vi "TM process commands.vi"(7 "Array in":T1[](array[typedef]) {"Time stamp" format="%<%H:%M:%S\n%Y/%m/%d>T"}, 8 "error in (no error)":errorcluster, 9 "Data":variant, 10 "Command":T2, 11 "Temperature monitor status in":T3 {"Last update" format="%<%H:%M:%S\n%y/%m/%d>T"}) -> (0 "error out":errorcluster, 1 "End?":bool, 2 "Array out":T1[](array[typedef]) {"Time stamp" format="%<%H:%M:%S\n%Y/%m/%d>T"}, 3 "Temperature monitor status out":T3 {"Last update" format="%<%H:%M:%S\n%y/%m/%d>T"})   [LabVIEW 2021, in "Temperature monitor.lvlib"]
uses:
  Temperature monitor.lvlib
  Typedefs/TM_status.ctl
  <userlib>/MatS Libs/MatS Mailman/TypeDefs/Mailbox ref.ctl
  Typedefs/TM_commands.ctl
  Typedefs/TM_sensors.ctl
  <userlib>/MatS Libs/MatS Libs.lvlib
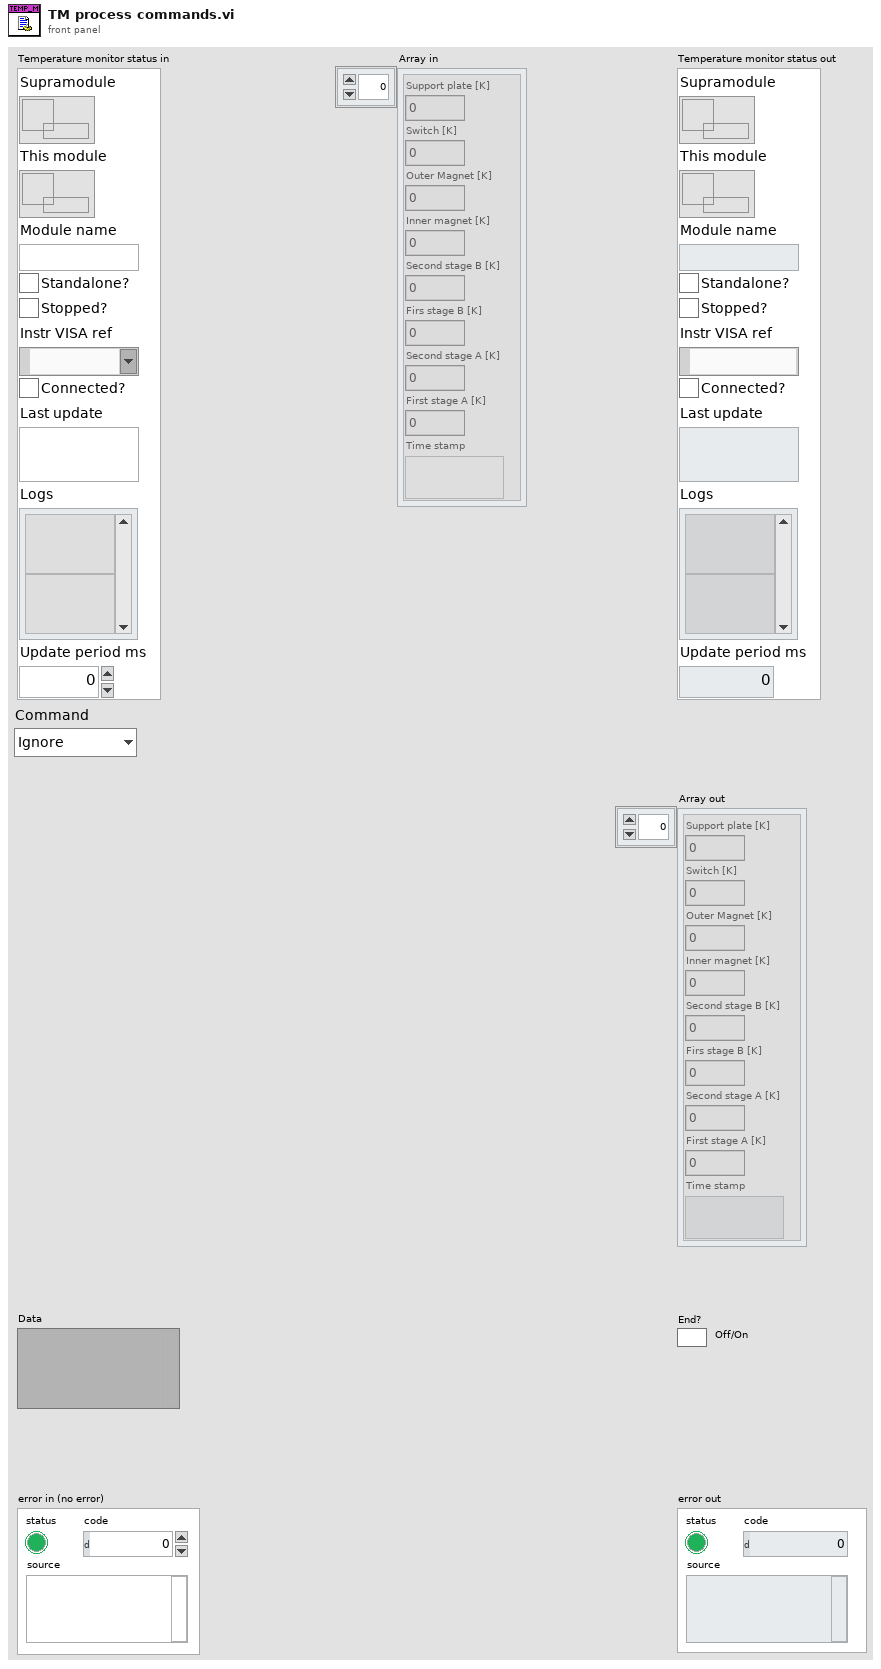
[diagram p1: front panel]
types:
  T1 = typedef "Temperature monitor.lvlib/TM_sensors.ctl" = cluster{"Support plate [K]":dbl, "Switch [K]":dbl, "Outer Magnet [K]":dbl, "Inner magnet [K]":dbl, "Second stage B [K]":dbl, "Firs stage B [K]":dbl, "Second stage A [K]":dbl, "First stage A [K]":dbl, "Time stamp":timestamp}
  T2 = typedef "Temperature monitor.lvlib/TM_commands.ctl" = enum16{"Ignore", "Log", "Connect", "Set timeout", "Update", "Disconnect", "End"}
  T3 = typedef "Temperature monitor.lvlib/TM_status.ctl" = cluster{"Supramodule":T4, "This module":T4, "Module name":string, "Standalone?":bool, "Stopped?":bool, "Instr VISA ref":refnum<visa-resource-name>, "Connected?":bool, "Last update":timestamp, "Logs":string[], "Update period ms":u32}
  T4 = typedef "MatS Libs.lvlib/Mailbox ref.ctl" = refnum<queue>
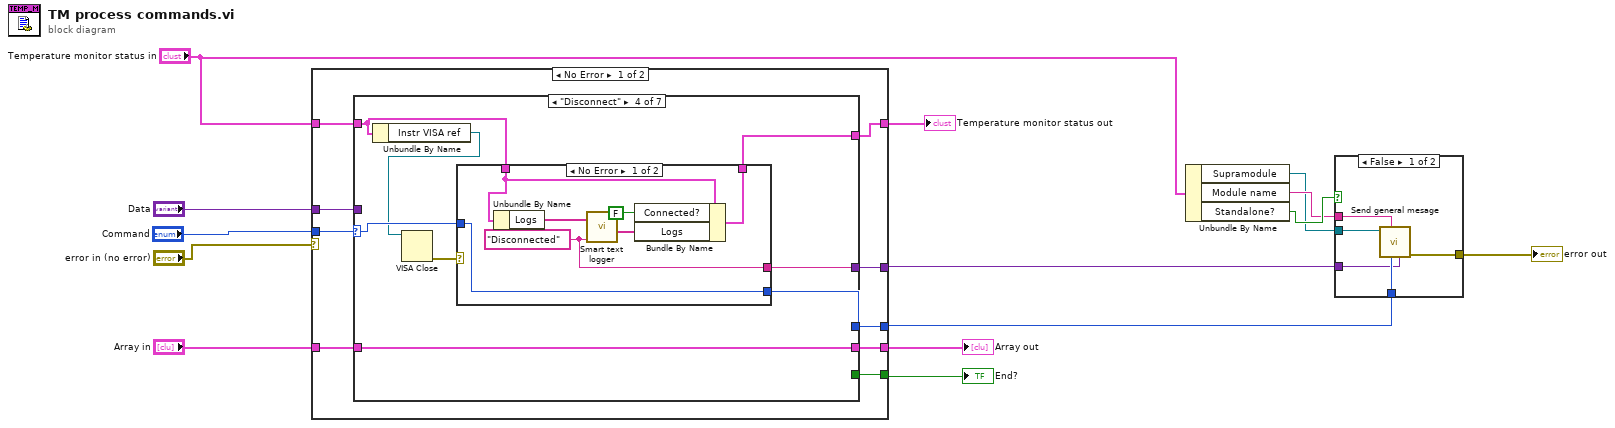
[diagram p0: block diagram]
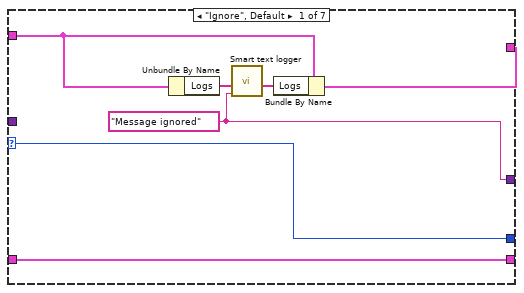
[diagram p2: hidden frame]
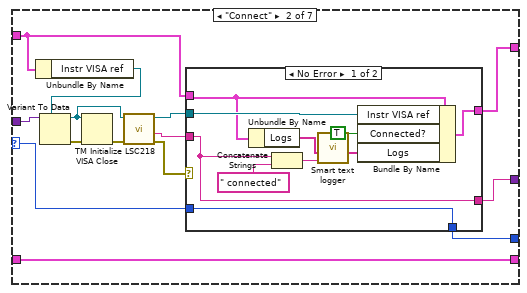
[diagram p3: hidden frame]
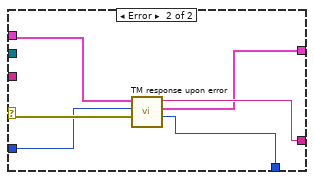
[diagram p4: hidden frame]
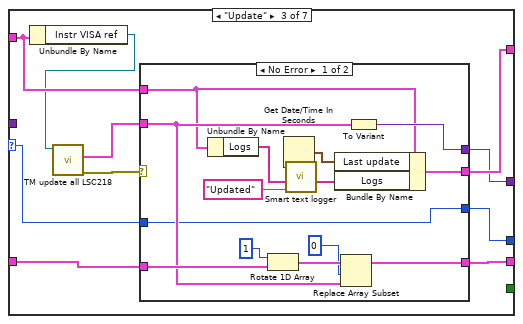
[diagram p5: hidden frame]
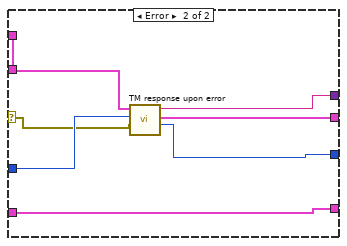
[diagram p6: hidden frame]
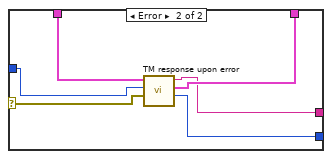
[diagram p7: hidden frame]
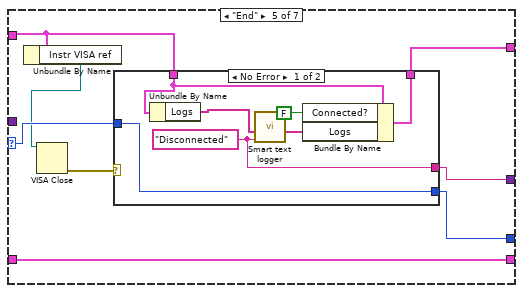
[diagram p8: hidden frame]
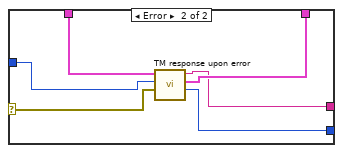
[diagram p9: hidden frame]
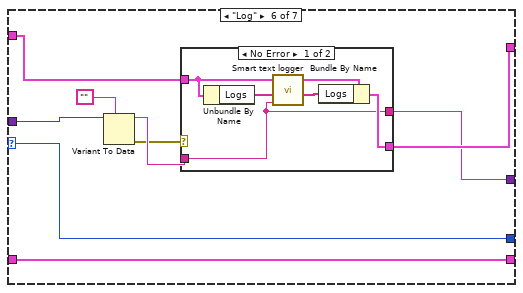
[diagram p10: hidden frame]
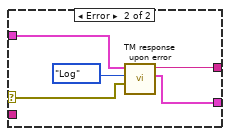
[diagram p11: hidden frame]
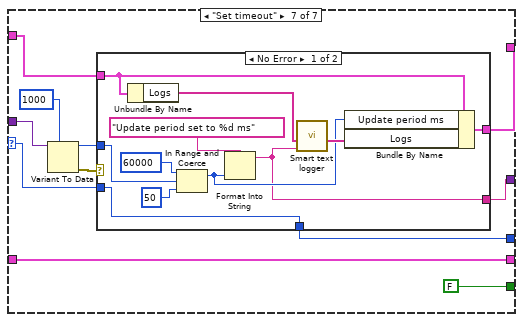
[diagram p12: hidden frame]
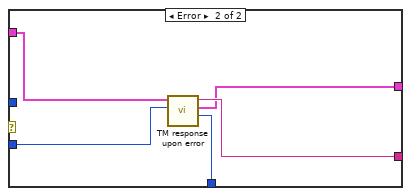
[diagram p13: hidden frame]
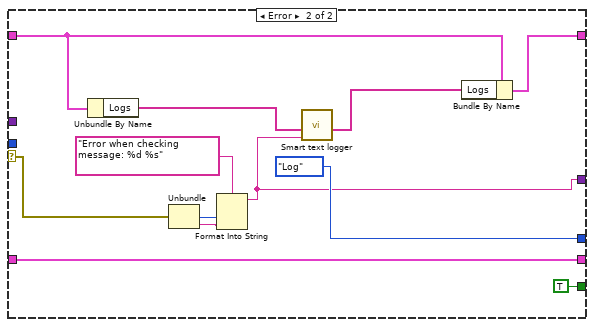
[diagram p14: hidden frame]
diagram:
  n1 = case shown="No Error" "error in (no error)" {
    selector: "error in (no error)" -> [_ w184]
    tunnel: "Temperature monitor status in" -> [w23 w183]
    tunnel: [w22 w182] -> w9
    tunnel: [w21 TRUE] -> w8
    tunnel: "Data" -> [w20 _]
    tunnel: [w19 w180] -> w6
    tunnel: "Array in" -> [w18 w180]
    tunnel: "Command" -> [w17 _]
    tunnel: [w16 TM_commands."Log" ("Command")] -> w3
    tunnel: [w15 w185] -> w2
    frame No Error {
      n2 = case shown="\"Disconnect\"" w17 {
        selector: w17 -> [w25 w33 w63 w96 w117 w138 w154]
        tunnel: w18 -> [w30 w44 w68 w99 w120 w142 w163]
        tunnel: [w30 w44 w67 w99 w120 w142 w163] -> w19
        tunnel: [_ _ _ _ _ _ FALSE] -> w21
        tunnel: w20 -> [_ w40 _ _ _ w140 w160]
        tunnel: [w28 w39 w69 w97 w119 w139 w158] -> w22
        tunnel: w23 -> [w27 w32 w62 w93 w114 w136 w157]
        tunnel: [w25 w34 w66 w95 w115 w138 w153] -> w16
        tunnel: [w24 w35 w64 w94 w116 w135 w155] -> w15
        frame "Ignore", Default {
          w24 = "Message ignored" ("Message")
          n3 = Unbundle By Name(w27) -> ("Logs"=w26:string[])
          n4 = call <userlib>:"Smart text logger.vi"("Message"=w24, "Logs in"=w26) -> ("Logs out"=w29:string[])  [unwired: 9 in]
          n5 = Bundle By Name(cluster=w27, "Logs"=w29) -> (w28:T3)
        }
        frame "Connect" {
          n6 = Unbundle By Name(w32) -> ("Instr VISA ref"=w31:refnum<visa-resource-name>)
          n7 = Variant To Data(type=w31, Variant=w40) -> (data=w41:refnum<visa-resource-name>, error out=w43:errorcluster)  [unwired: 1 in]
          n8 = VISA Close(VISA resource name=w41, error in (no error)=w43) -> (error out=w42:errorcluster)
          n9 = call "TM Initialize LSC218.vi"("error in (no error)"=w42, "VISA Refnum in"=w41) -> ("error out"=w37:errorcluster, "Instr Model Number"=w36:string, "VISA Refnum out"=w38:refnum<visa-resource-name>)  [unwired: 6 in, 1 out]
          n10 = case shown="No Error" w37 {
            selector: w37 -> [_ w59]
            tunnel: [w54 w55] -> w39
            tunnel: w38 -> [w53 _]
            tunnel: w32 -> [w48 w60]
            tunnel: w36 -> [w46 _]
            tunnel: [w46 w56] -> w35
            tunnel: [w45 w57] -> w34
            tunnel: w33 -> [w45 w58]
            frame No Error {
              n11 = Unbundle By Name(w48) -> ("Logs"=w47:string[])
              n12 = Concatenate Strings(w46, " connected" ("string")) -> (w52:string)
              n13 = call <userlib>:"Smart text logger.vi"("Message"=w52, "Logs in"=w47) -> ("Logs out"=w50:string[])  [unwired: 9 in]
              n14 = Bundle By Name(cluster=w48, "Instr VISA ref"=w53, "Connected?"=TRUE, "Logs"=w50) -> (w54:T3)
            }
            frame Error {
              n15 = call "TM response upon error.vi"("error in (no error)"=w59, "Command"=w58, "Temperature monitor status in in"=w60) -> ("Cmd out"=w57:T2, "Temperature monitor status out"=w55:T3, "Text message"=w56:string)  [unwired: 5 in, 1 out]
            }
          }
        }
        frame "Update" {
          n16 = Unbundle By Name(w62) -> ("Instr VISA ref"=w61:refnum<visa-resource-name>)
          n17 = call "TM update all LSC218.vi"("VISA Refnum in"=w61) -> ("error out"=w70:errorcluster, "LSC218 sensors"=w65:T1)  [unwired: 8 in, 1 out]
          n18 = case shown="No Error" w70 {
            selector: w70 -> [_ w85]
            tunnel: w62 -> [w72 w91]
            tunnel: [w83 w90] -> w69
            tunnel: w65 -> [w75 _]
            tunnel: w68 -> [w80 w89]
            tunnel: [w79 w89] -> w67
            tunnel: [w73 w87] -> w66
            tunnel: [w76 w88] -> w64
            tunnel: w63 -> [w73 w86]
            frame No Error {
              n19 = Unbundle By Name(w72) -> ("Logs"=w71:string[])
              n20 = Rotate 1D Array(1:w80, 2:1 ("n")) -> (0:w82:T1[])
              n21 = Get Date/Time In Seconds() -> (seconds since 1Jan1904=w84:timestamp)
              n22 = call <userlib>:"Smart text logger.vi"("Message"="Updated", "Logs in"=w71) -> ("Logs out"=w77:string[])  [unwired: 9 in]
              n23 = Bundle By Name(cluster=w72, "Last update"=w84, "Logs"=w77) -> (w83:T3)
              n24 = Replace Array Subset(array=w82, new element=w75, index=0) -> (w79:T1[])
              n25 = To Variant(anything=w75) -> (Variant=w76:variant)
            }
            frame Error {
              n26 = call "TM response upon error.vi"("error in (no error)"=w85, "Command"=w86, "Temperature monitor status in in"=w91) -> ("Cmd out"=w87:T2, "Temperature monitor status out"=w90:T3, "Text message"=w88:string)  [unwired: 5 in, 1 out]
            }
          }
        }
        frame "Disconnect" {
          n27 = Unbundle By Name(w93) -> ("Instr VISA ref"=w92:refnum<visa-resource-name>)
          n28 = VISA Close(VISA resource name=w92) -> (error out=w98:errorcluster)  [unwired: 1 in]
          n29 = case shown="No Error" w98 {
            selector: w98 -> [_ w107]
            tunnel: w93 -> [w101 w112]
            tunnel: [w105 w111] -> w97
            tunnel: w96 -> [w103 w108]
            tunnel: [w103 w109] -> w95
            tunnel: [w102 w110] -> w94
            frame No Error {
              w102 = "Disconnected" ("Message")
              n30 = Unbundle By Name(w101) -> ("Logs"=w100:string[])
              n31 = call <userlib>:"Smart text logger.vi"("Message"=w102, "Logs in"=w100) -> ("Logs out"=w104:string[])  [unwired: 9 in]
              n32 = Bundle By Name(cluster=w101, "Connected?"=FALSE, "Logs"=w104) -> (w105:T3)
            }
            frame Error {
              n33 = call "TM response upon error.vi"("error in (no error)"=w107, "Command"=w108, "Temperature monitor status in in"=w112) -> ("Cmd out"=w109:T2, "Temperature monitor status out"=w111:T3, "Text message"=w110:string)  [unwired: 5 in, 1 out]
            }
          }
        }
        frame "End" {
          n34 = Unbundle By Name(w114) -> ("Instr VISA ref"=w113:refnum<visa-resource-name>)
          n35 = VISA Close(VISA resource name=w113) -> (error out=w118:errorcluster)  [unwired: 1 in]
          n36 = case shown="No Error" w118 {
            selector: w118 -> [_ w128]
            tunnel: w114 -> [w121 w133]
            tunnel: [w126 w132] -> w119
            tunnel: w117 -> [w124 w129]
            tunnel: [w124 w130] -> w115
            tunnel: [w123 w131] -> w116
            frame No Error {
              w123 = "Disconnected" ("Message")
              n37 = Unbundle By Name(w121) -> ("Logs"=w122:string[])
              n38 = call <userlib>:"Smart text logger.vi"("Message"=w123, "Logs in"=w122) -> ("Logs out"=w125:string[])  [unwired: 9 in]
              n39 = Bundle By Name(cluster=w121, "Connected?"=FALSE, "Logs"=w125) -> (w126:T3)
            }
            frame Error {
              n40 = call "TM response upon error.vi"("error in (no error)"=w128, "Command"=w129, "Temperature monitor status in in"=w133) -> ("Cmd out"=w130:T2, "Temperature monitor status out"=w132:T3, "Text message"=w131:string)  [unwired: 5 in, 1 out]
            }
          }
        }
        frame "Log" {
          n41 = Variant To Data(type="", Variant=w140) -> (data=w137:string, error out=w134:errorcluster)  [unwired: 1 in]
          n42 = case shown="No Error" w134 {
            selector: w134 -> [_ w149]
            tunnel: [w146 w151] -> w139
            tunnel: w137 -> [w143 _]
            tunnel: w136 -> [w145 w152]
            tunnel: [w143 w150] -> w135
            frame No Error {
              n43 = Unbundle By Name(w145) -> ("Logs"=w144:string[])
              n44 = call <userlib>:"Smart text logger.vi"("Message"=w143, "Logs in"=w144) -> ("Logs out"=w147:string[])  [unwired: 9 in]
              n45 = Bundle By Name(cluster=w145, "Logs"=w147) -> (w146:T3)
            }
            frame Error {
              n46 = call "TM response upon error.vi"("error in (no error)"=w149, "Command"=TM_commands."Log", "Temperature monitor status in in"=w152) -> ("Temperature monitor status out"=w151:T3, "Text message"=w150:string)  [unwired: 5 in, 2 out]
            }
          }
        }
        frame "Set timeout" {
          n47 = Variant To Data(type=1000 ("timeout ms"), Variant=w160) -> (data=w159:i32, error out=w156:errorcluster)  [unwired: 1 in]
          n48 = case shown="No Error" w156 {
            tunnel: w159 -> [w174 _]
            tunnel: [w168 w176] -> w158
            tunnel: w157 -> [w166 w179]
            tunnel: w154 -> [w164 w178]
            tunnel: [w167 w177] -> w155
            tunnel: [w164 w175] -> w153
            frame No Error {
              n49 = Unbundle By Name(w166) -> ("Logs"=w165:string[])
              n50 = In Range and Coerce(upper limit=60000, x=w174, lower limit=50) -> (coerced(x)=w169:i32)  [unwired: 1 out]
              n51 = Format Into String(format string="Update period set to %d ms", w169) -> (resulting string=w167:string)  [unwired: 2 in, 1 out]
              n52 = call <userlib>:"Smart text logger.vi"("Message"=w167, "Logs in"=w165) -> ("Logs out"=w171:string[])  [unwired: 9 in]
              n53 = Bundle By Name(cluster=w166, "Update period ms"=w169, "Logs"=w171) -> (w168:T3)
            }
            frame Error {
              n54 = call "TM response upon error.vi"("Command"=w178, "Temperature monitor status in in"=w179) -> ("Cmd out"=w175:T2, "Temperature monitor status out"=w176:T3, "Text message"=w177:string)  [unwired: 6 in, 1 out]
            }
          }
        }
      }
    }
    frame Error {
      n55 = Unbundle By Name(w183) -> ("Logs"=w187:string[])
      n56 = Unbundle(w184) -> ("code"=w190:i32, "source"=w189:string)  [unwired: 1 out]
      n57 = Format Into String(format string="Error when checking message: %d %s", w190, w189) -> (resulting string=w185:string)  [unwired: 2 in, 1 out]
      n58 = call <userlib>:"Smart text logger.vi"("Message"=w185, "Logs in"=w187) -> ("Logs out"=w181:string[])  [unwired: 9 in]
      n59 = Bundle By Name(cluster=w183, "Logs"=w181) -> (w182:T3)
    }
  }
  "Temperature monitor status out" <- w9
  "End?" <- w8
  "Array out" <- w6
  n60 = Unbundle By Name("Temperature monitor status in") -> ("Supramodule"=w11:T4, "Module name"=w12:string, "Standalone?"=w13:bool)
  n61 = case shown="False" w13 {
    tunnel: w11 -> [w196 _]
    tunnel: [w195 _] -> w10
    tunnel: w12 -> [w194 _]
    tunnel: w3 -> [w193 _]
    tunnel: w2 -> [w192 _]
    frame False {
      n62 = call <userlib>:"Send general mesage.vi"("Content"=w192, "Topic"=w193, "Sender"=w194, "Mailbox ref in"=w196) -> ("error out"=w195:errorcluster)  [unwired: 5 in, 2 out]
    }
    frame True {
    }
  }
  "error out" <- w10
